vi "Update Graphs_v1.35.vi"(0 "ERD_Always Show":T3, 1 "Select Graph":T2, 3 "appended array":refnum<vi>[](array[refnum]), 4 "ERD Graph  Ind 2":T1, 5 "Error In":errorcluster) -> (11 "ERD 1":dbl(graph), 12 "Motor Current":dbl(graph), 13 "ERD 2":dbl(graph), 14 "Temp":dbl(graph), 15 "Basket Speed":u16(graph), 16 "ERD 3":dbl(graph), 17 "Tub Gallons":dbl(graph), 18 "Pressure 3":dbl(graph), 19 "Error Out":errorcluster)   [LabVIEW 2014]
doc: "This VI displays (makes visable) the corresponding graph based on user selection, as well as updates the values of the graphs with current data."
uses:
  type defs/ERD_Always_Show.ctl
  type defs/Select Graph.ctl
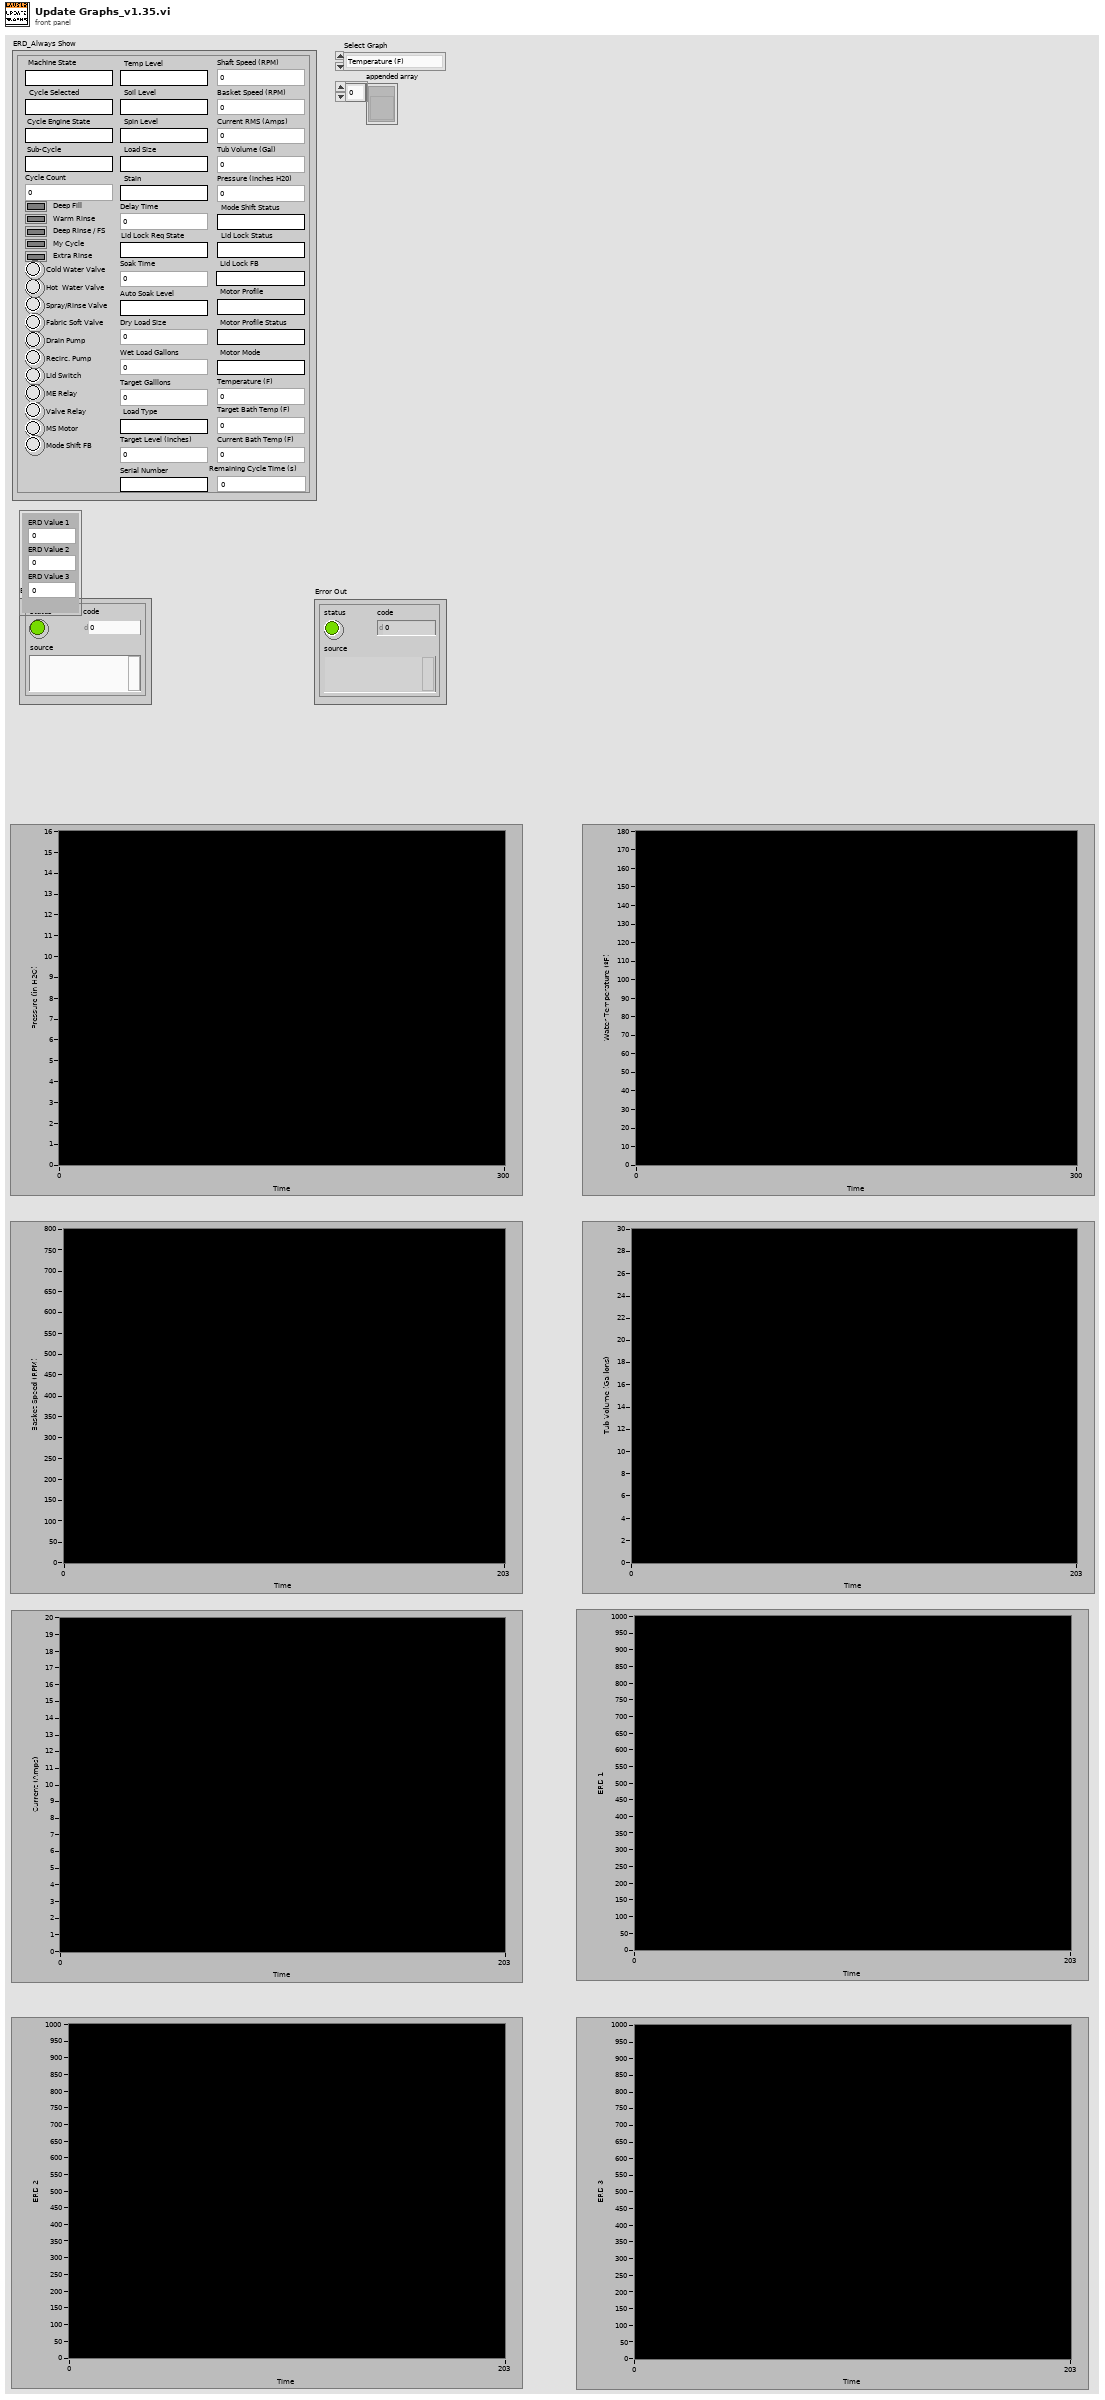
[diagram p1: front panel]
types:
  T1 = cluster{"ERD Value 1":dbl, "ERD Value 2":dbl, "ERD Value 3":dbl}
  T2 = typedef "Select Graph.ctl" = enum16{"Temperature (F)", "Basket Speed (RPM)", "Tub Volume (Gal)", "Pressure (in H2O)", "Current RMS (Amps)", "ERD 1", "ERD 2", "ERD 3"}
  T3 = typedef "ERD_Always_Show.ctl" = cluster{"Basket Speed (RPM)":u16, "Machine State":string, "Tub Volume (Gal)":dbl, "Pressure (inches H20)":dbl, "Lid Switch ":bool, "Current RMS (Amps)":dbl, "Cycle Selected":string, "Lid Lock Status":string, "Mode Shift Status":string, "Spray/Rinse Valve":bool, "Fabric Soft Valve":bool, "Drain Pump":bool, "Recirc. Pump":bool, "Cycle Engine State":string, "Hot  Water Valve":bool, "Cold Water Valve":bool, "Motor Profile":string, "Motor Profile Status":string, "Motor Mode":string, "ME Relay":bool, "Cycle Count":u32, "Deep Rinse / FS":bool, "My Cycle":bool, "Soil Level":string, "Spin Level":string, "Stain":string, "Temp Level":string, "Load Size":string, "Delay Time":u16, "Soak Time":u16, "Deep Fill":bool, "Warm Rinse":bool, "Auto Soak Level":string, "Extra Rinse":bool, "Wet Load Gallons":dbl, "Target Galllons":dbl, "Sub-Cycle":string, "Load Type":string, "Target Level (inches)":u32, "Valve Relay":bool, "Dry Load Size":dbl, "Shaft Speed (RPM) ":u16, "MS Motor":bool, "Mode Shift FB":bool, "Target Bath Temp (F)":dbl, "Temperature (F)":dbl, "Current Bath Temp (F)":dbl, "Lid Lock FB":string, "Lid Lock Req State":string, "Remaining Cycle Time (s)":dbl, "Serial Number":string}
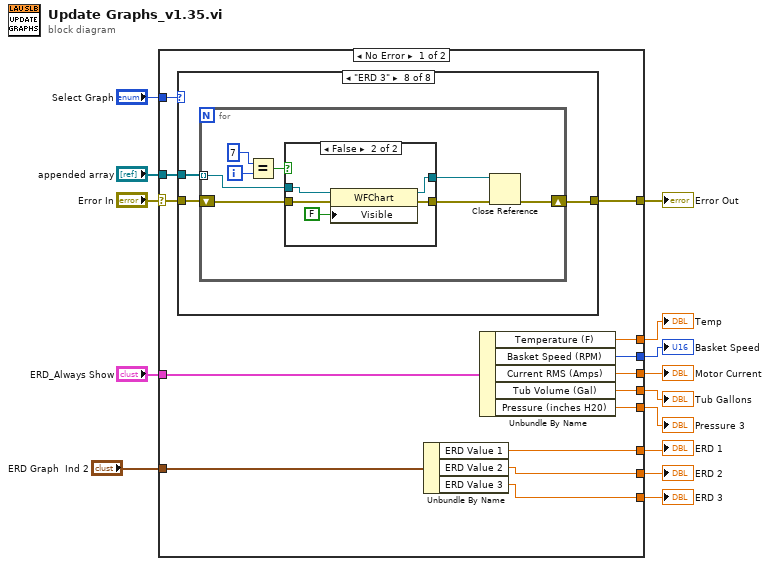
[diagram p0: block diagram]
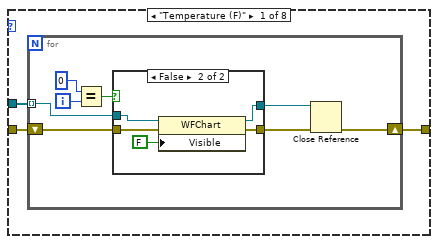
[diagram p2: hidden frame]
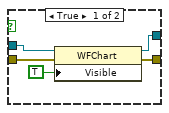
[diagram p3: hidden frame]
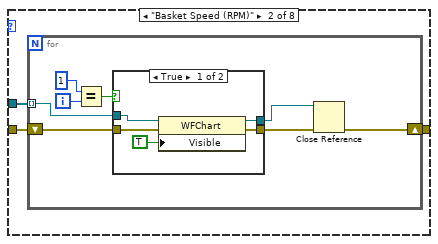
[diagram p4: hidden frame]
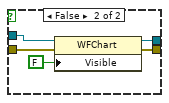
[diagram p5: hidden frame]
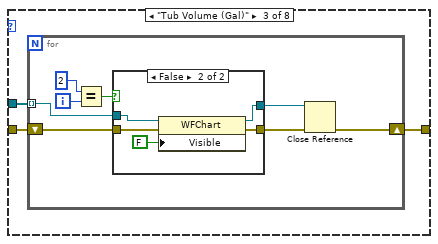
[diagram p6: hidden frame]
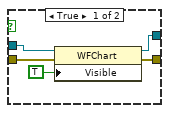
[diagram p7: hidden frame]
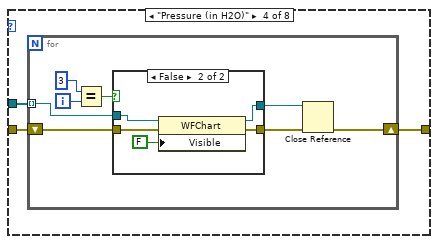
[diagram p8: hidden frame]
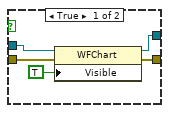
[diagram p9: hidden frame]
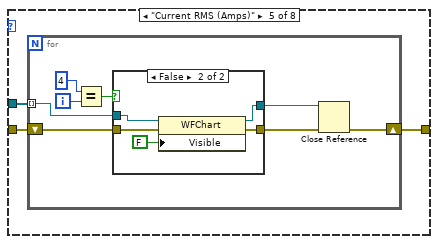
[diagram p10: hidden frame]
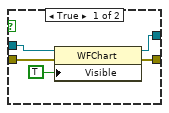
[diagram p11: hidden frame]
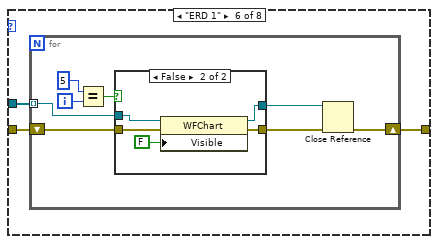
[diagram p12: hidden frame]
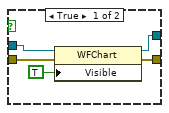
[diagram p13: hidden frame]
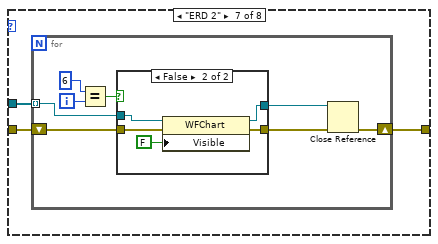
[diagram p14: hidden frame]
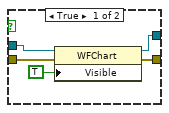
[diagram p15: hidden frame]
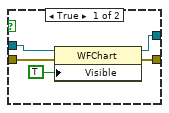
[diagram p16: hidden frame]
diagram:
  n1 = case shown="No Error" "Error In" {
    selector: "Error In" -> [w25 w197]
    tunnel: [w24 w197] -> w13
    tunnel: "ERD_Always Show" -> [w28 _]
    tunnel: "appended array" -> [w26 _]
    tunnel: "Select Graph" -> [w27 _]
    tunnel: [w23 _] -> w9
    tunnel: [w22 _] -> w8
    tunnel: [w21 _] -> w7
    tunnel: [w20 _] -> w6
    tunnel: [w19 _] -> w5
    tunnel: "ERD Graph  Ind 2" -> [w18 _]
    tunnel: [w17 _] -> w3
    tunnel: [w16 _] -> w2
    tunnel: [w15 _] -> w1
    frame No Error {
      n2 = case shown="\"ERD 3\"" w27 {
        tunnel: w26 -> [w31 w52 w73 w94 w114 w135 w157 w176]
        tunnel: w25 -> [w30 w51 w72 w93 w115 w136 w156 w178]
        tunnel: [w29 w50 w71 w92 w113 w134 w155 w177] -> w24
        frame "Temperature (F)" {
          n3 = for {
            tunnel: w31 -> [w39] mode=indexing
            shift-right: [w33] -> w29
            shift-left: w30 -> [w38]
            i -> [w37]
            n4 = Equal?(x=0 ("index"), y=w37) -> (x = y?=w35:bool)
            n5 = case shown="False" w35 {
              tunnel: w39 -> [w44 w49]
              tunnel: w38 -> [w42 w47]
              tunnel: [w41 w46] -> w34
              tunnel: [w40 w45] -> w32
              frame True {
                n6 = property class="WFChart"(reference=w44, error in=w42, "Visible"=TRUE) -> (reference out=w40:refnum<vi>, error out=w41:errorcluster)
              }
              frame False {
                n7 = property class="WFChart"(reference=w49, error in=w47, "Visible"=FALSE) -> (reference out=w45:refnum<vi>, error out=w46:errorcluster)
              }
            }
            n8 = Close Reference(reference=w32, error in (no error)=w34) -> (error out=w33:errorcluster)
          }
        }
        frame "Basket Speed (RPM)" {
          n9 = for {
            tunnel: w52 -> [w60] mode=indexing
            shift-right: [w53] -> w50
            shift-left: w51 -> [w59]
            i -> [w58]
            n10 = Equal?(x=1 ("index"), y=w58) -> (x = y?=w56:bool)
            n11 = case shown="True" w56 {
              tunnel: w60 -> [w65 w70]
              tunnel: w59 -> [w63 w68]
              tunnel: [w62 w67] -> w54
              tunnel: [w61 w66] -> w55
              frame True {
                n12 = property class="WFChart"(reference=w65, error in=w63, "Visible"=TRUE) -> (reference out=w61:refnum<vi>, error out=w62:errorcluster)
              }
              frame False {
                n13 = property class="WFChart"(reference=w70, error in=w68, "Visible"=FALSE) -> (reference out=w66:refnum<vi>, error out=w67:errorcluster)
              }
            }
            n14 = Close Reference(reference=w55, error in (no error)=w54) -> (error out=w53:errorcluster)
          }
        }
        frame "Tub Volume (Gal)" {
          n15 = for {
            tunnel: w73 -> [w81] mode=indexing
            shift-right: [w75] -> w71
            shift-left: w72 -> [w80]
            i -> [w79]
            n16 = Equal?(x=2 ("index"), y=w79) -> (x = y?=w77:bool)
            n17 = case shown="False" w77 {
              tunnel: w81 -> [w86 w91]
              tunnel: w80 -> [w84 w89]
              tunnel: [w83 w88] -> w76
              tunnel: [w82 w87] -> w74
              frame True {
                n18 = property class="WFChart"(reference=w86, error in=w84, "Visible"=TRUE) -> (reference out=w82:refnum<vi>, error out=w83:errorcluster)
              }
              frame False {
                n19 = property class="WFChart"(reference=w91, error in=w89, "Visible"=FALSE) -> (reference out=w87:refnum<vi>, error out=w88:errorcluster)
              }
            }
            n20 = Close Reference(reference=w74, error in (no error)=w76) -> (error out=w75:errorcluster)
          }
        }
        frame "Pressure (in H2O)" {
          n21 = for {
            tunnel: w94 -> [w102] mode=indexing
            shift-right: [w96] -> w92
            shift-left: w93 -> [w101]
            i -> [w100]
            n22 = Equal?(x=3 ("index"), y=w100) -> (x = y?=w98:bool)
            n23 = case shown="False" w98 {
              tunnel: w102 -> [w107 w112]
              tunnel: w101 -> [w105 w110]
              tunnel: [w104 w109] -> w97
              tunnel: [w103 w108] -> w95
              frame True {
                n24 = property class="WFChart"(reference=w107, error in=w105, "Visible"=TRUE) -> (reference out=w103:refnum<vi>, error out=w104:errorcluster)
              }
              frame False {
                n25 = property class="WFChart"(reference=w112, error in=w110, "Visible"=FALSE) -> (reference out=w108:refnum<vi>, error out=w109:errorcluster)
              }
            }
            n26 = Close Reference(reference=w95, error in (no error)=w97) -> (error out=w96:errorcluster)
          }
        }
        frame "Current RMS (Amps)" {
          n27 = for {
            tunnel: w114 -> [w123] mode=indexing
            shift-right: [w117] -> w113
            shift-left: w115 -> [w122]
            i -> [w121]
            n28 = Equal?(x=4 ("index"), y=w121) -> (x = y?=w119:bool)
            n29 = case shown="False" w119 {
              tunnel: w123 -> [w128 w133]
              tunnel: w122 -> [w126 w131]
              tunnel: [w125 w130] -> w118
              tunnel: [w124 w129] -> w116
              frame True {
                n30 = property class="WFChart"(reference=w128, error in=w126, "Visible"=TRUE) -> (reference out=w124:refnum<vi>, error out=w125:errorcluster)
              }
              frame False {
                n31 = property class="WFChart"(reference=w133, error in=w131, "Visible"=FALSE) -> (reference out=w129:refnum<vi>, error out=w130:errorcluster)
              }
            }
            n32 = Close Reference(reference=w116, error in (no error)=w118) -> (error out=w117:errorcluster)
          }
        }
        frame "ERD 1" {
          n33 = for {
            tunnel: w135 -> [w144] mode=indexing
            shift-right: [w138] -> w134
            shift-left: w136 -> [w143]
            i -> [w142]
            n34 = Equal?(x=5 ("index"), y=w142) -> (x = y?=w140:bool)
            n35 = case shown="False" w140 {
              tunnel: w144 -> [w149 w154]
              tunnel: w143 -> [w147 w152]
              tunnel: [w146 w151] -> w139
              tunnel: [w145 w150] -> w137
              frame True {
                n36 = property class="WFChart"(reference=w149, error in=w147, "Visible"=TRUE) -> (reference out=w145:refnum<vi>, error out=w146:errorcluster)
              }
              frame False {
                n37 = property class="WFChart"(reference=w154, error in=w152, "Visible"=FALSE) -> (reference out=w150:refnum<vi>, error out=w151:errorcluster)
              }
            }
            n38 = Close Reference(reference=w137, error in (no error)=w139) -> (error out=w138:errorcluster)
          }
        }
        frame "ERD 2" {
          n39 = for {
            tunnel: w157 -> [w165] mode=indexing
            shift-right: [w159] -> w155
            shift-left: w156 -> [w164]
            i -> [w163]
            n40 = Equal?(x=6 ("index"), y=w163) -> (x = y?=w161:bool)
            n41 = case shown="False" w161 {
              tunnel: w165 -> [w170 w175]
              tunnel: w164 -> [w168 w173]
              tunnel: [w167 w172] -> w160
              tunnel: [w166 w171] -> w158
              frame True {
                n42 = property class="WFChart"(reference=w170, error in=w168, "Visible"=TRUE) -> (reference out=w166:refnum<vi>, error out=w167:errorcluster)
              }
              frame False {
                n43 = property class="WFChart"(reference=w175, error in=w173, "Visible"=FALSE) -> (reference out=w171:refnum<vi>, error out=w172:errorcluster)
              }
            }
            n44 = Close Reference(reference=w158, error in (no error)=w160) -> (error out=w159:errorcluster)
          }
        }
        frame "ERD 3" {
          n45 = for {
            tunnel: w176 -> [w186] mode=indexing
            shift-right: [w180] -> w177
            shift-left: w178 -> [w185]
            i -> [w184]
            n46 = Equal?(x=7 ("index"), y=w184) -> (x = y?=w182:bool)
            n47 = case shown="False" w182 {
              tunnel: w186 -> [w191 w196]
              tunnel: w185 -> [w189 w194]
              tunnel: [w188 w193] -> w181
              tunnel: [w187 w192] -> w179
              frame True {
                n48 = property class="WFChart"(reference=w191, error in=w189, "Visible"=TRUE) -> (reference out=w187:refnum<vi>, error out=w188:errorcluster)
              }
              frame False {
                n49 = property class="WFChart"(reference=w196, error in=w194, "Visible"=FALSE) -> (reference out=w192:refnum<vi>, error out=w193:errorcluster)
              }
            }
            n50 = Close Reference(reference=w179, error in (no error)=w181) -> (error out=w180:errorcluster)
          }
        }
      }
      n51 = Unbundle By Name(w18) -> ("ERD Value 1"=w17:dbl, "ERD Value 2"=w16:dbl, "ERD Value 3"=w15:dbl)
      n52 = Unbundle By Name(w28) -> ("Temperature (F)"=w23:dbl, "Basket Speed (RPM)"=w22:u16, "Current RMS (Amps)"=w21:dbl, "Tub Volume (Gal)"=w20:dbl, "Pressure (inches H20)"=w19:dbl)
    }
    frame Error {
    }
  }
  "Error Out" <- w13
  "Temp" <- w9
  "Basket Speed" <- w8
  "Motor Current" <- w7
  "Tub Gallons" <- w6
  "Pressure 3" <- w5
  "ERD 1" <- w3
  "ERD 2" <- w2
  "ERD 3" <- w1
